vi "VL53L0X_GetDeviceInfo.vi"(11 "REV2mDistanceSensorDevRef":T2) -> (2 "DeviceInfo":T1, 3 "REV2mDistanceSensorDevRef Out":T2)   [LabVIEW 2019, in "DistanceSensorDriver.lvlib"]
uses:
  DistanceSensorDriver.lvlib
  Typedef/REV2mDistanceSensorDevRef.ctl
  Typedef/Ports.ctl
  Typedef/VL53L0X_DeviceInfo_t.ctl
panel:
  in  "VL53L0X_DeviceInfo_t":T1
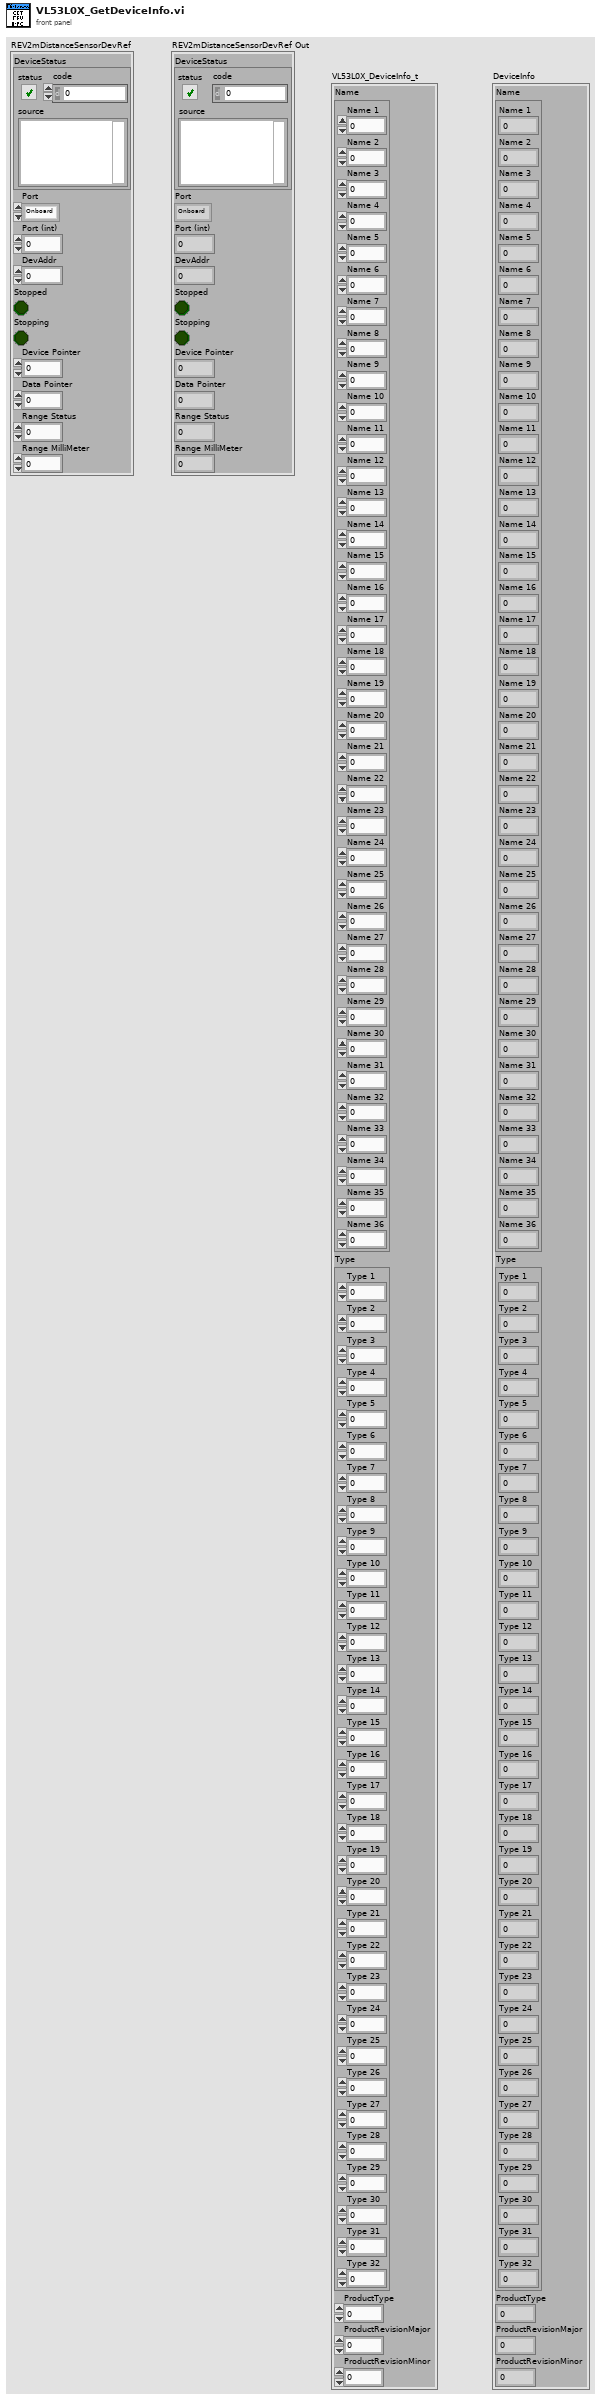
[diagram p1: front panel]
types:
  T1 = typedef "DistanceSensorDriver.lvlib/VL53L0X_DeviceInfo_t.ctl" = cluster{"Name":cluster{"Name 1":i8, "Name 2":i8, "Name 3":i8, "Name 4":i8, "Name 5":i8, "Name 6":i8, "Name 7":i8, "Name 8":i8, "Name 9":i8, "Name 10":i8, "Name 11":i8, "Name 12":i8, "Name 13":i8, "Name 14":i8, "Name 15":i8, "Name 16":i8, "Name 17":i8, "Name 18":i8, "Name 19":i8, "Name 20":i8, "Name 21":i8, "Name 22":i8, "Name 23":i8, "Name 24":i8, "Name 25":i8, "Name 26":i8, "Name 27":i8, "Name 28":i8, "Name 29":i8, "Name 30":i8, "Name 31":i8, "Name 32":i8, "Name 33":i8, "Name 34":i8, "Name 35":i8, "Name 36":i8}, "Type":cluster{"Type 1":i8, "Type 2":i8, "Type 3":i8, "Type 4":i8, "Type 5":i8, "Type 6":i8, "Type 7":i8, "Type 8":i8, "Type 9":i8, "Type 10":i8, "Type 11":i8, "Type 12":i8, "Type 13":i8, "Type 14":i8, "Type 15":i8, "Type 16":i8, "Type 17":i8, "Type 18":i8, "Type 19":i8, "Type 20":i8, "Type 21":i8, "Type 22":i8, "Type 23":i8, "Type 24":i8, "Type 25":i8, "Type 26":i8, "Type 27":i8, "Type 28":i8, "Type 29":i8, "Type 30":i8, "Type 31":i8, "Type 32":i8}, "ProductType":u8, "ProductRevisionMajor":u8, "ProductRevisionMinor":u8}
  T2 = typedef "DistanceSensorDriver.lvlib/REV2mDistanceSensorDevRef.ctl" = cluster{"DeviceStatus":errorcluster, "Port":T3, "Port (int)":i32, "DevAddr":i32, "Stopped":bool, "Stopping":bool, "Device Pointer":u64, "Data Pointer":u64, "Range Status":u8, "Range MilliMeter":u16}
  T3 = typedef "DistanceSensorDriver.lvlib/Ports.ctl" = enum32{"Onboard", "MXP"}
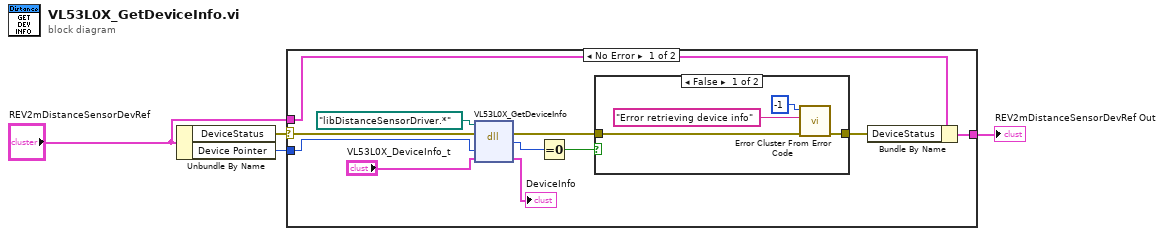
[diagram p0: block diagram]
diagram:
  n1 = Unbundle By Name("REV2mDistanceSensorDevRef") -> ("DeviceStatus"=w1:errorcluster, "Device Pointer"=w4:u64)
  n2 = case shown="No Error" w1 {
    selector: w1 -> [w5 _]
    tunnel: w4 -> [w10 _]
    tunnel: [w9 w21] -> w3
    tunnel: "REV2mDistanceSensorDevRef" -> [w8 w21]
    frame No Error {
      n3 = dll-call lib="?" fn="VL53L0X_GetDeviceInfo"(path in=path "libDistanceSensorDriver.*", error in=w5, "Dev"=w10, "DeviceInfo"="VL53L0X_DeviceInfo_t") -> (error out=w11:errorcluster, "Status"=w12:i32, "DeviceInfo"=→"DeviceInfo":T1)  [unwired: 2 in, 1 out]
      n4 = Equal To 0?(x=w12) -> (x = 0?=w15:bool)
      n5 = case shown="False" w15 {
        tunnel: w11 -> [w16 w20]
        tunnel: [w19 w20] -> w14
        frame False {
          n6 = call <vilib>:"Error Cluster From Error Code.vi"("error in (no error)"=w16, "error message (\"\")"="Error retrieving device info" ("error message (\"\")"), "error code (0)"=-1) -> ("error out"=w19:errorcluster)  [unwired: 6 in]
        }
        frame True {
        }
      }
      n7 = Bundle By Name(cluster=w8, "DeviceStatus"=w14) -> (w9:T2)
    }
    frame Error {
    }
  }
  "REV2mDistanceSensorDevRef Out" <- w3
